vi "PathToROI.vi"(10 "Path In":cluster{i32, i32}[](array[cluster])) -> (3 "ROI Out":T1)   [LabVIEW 2019]
doc: "Converts a path of pixels into a ROI"
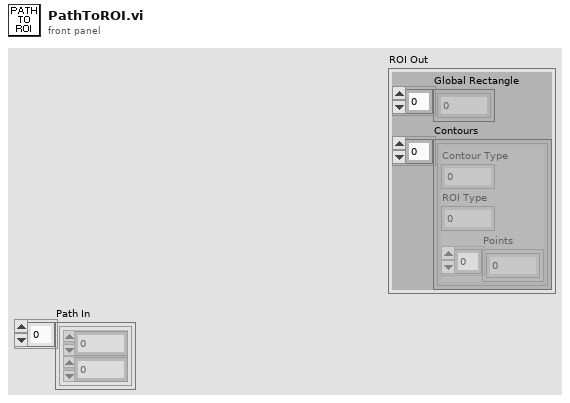
[diagram p1: front panel]
types:
  T1 = cluster{"Global Rectangle":i32[], "Contours":cluster{"Contour Type":u32, "ROI Type":u32, "Points":i32[]}[]}
  T2 = cluster{"Contour Type":u32, "ROI Type":u32, "Points":i32[]}[]
  T3 = cluster{"Contour Type":u32, "ROI Type":u32, "Points":i32[]}
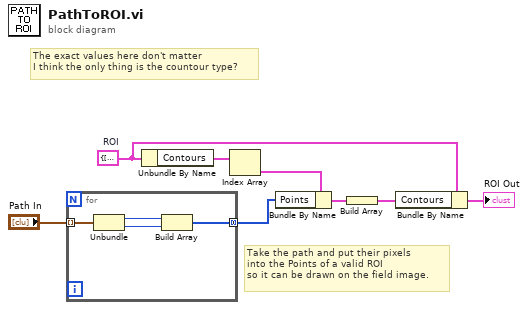
[diagram p0: block diagram]
diagram:
  w1 = T1 {"Global Rectangle"=[40, 76, 324, 119], "Contours"=[{"Contour Type"=0, "ROI Type"=10, "Points"=[40, 78, 202, 76, 323, 118]}]}  # ROI
  # "Take the path and put their pixels\ninto the Points of a valid ROI\nso it can be drawn on the field image."
  # "The exact values here don't matter\nI think the only thing is the countour type?"
  n1 = for {
    tunnel: [w10] -> w8 mode=concatenating
    tunnel: "Path In" -> [w9] mode=indexing
    n2 = Unbundle(w9) -> (w12:i32, w11:i32)
    n3 = Build Array(w12, w11) -> (w10:i32[])
  }
  n4 = Unbundle By Name(w1) -> ("Contours"=w4:T2)
  n5 = Index Array(array=w4) -> (element=w3:T3)  [unwired: 1 in]
  n6 = Bundle By Name(cluster=w3, "Points"=w8) -> (w6:T3)
  n7 = Build Array(w6) -> (w7:T2)
  n8 = Bundle By Name(cluster=w1, "Contours"=w7) -> (→"ROI Out":T1)
